vi "xxxx.vi"(8 "error in (no error)":errorcluster, 11 "Context Actor in":refnum<class "Context Actor.lvclass">) -> (0 "error out":errorcluster, 3 "Context Actor out":refnum<class "Context Actor.lvclass">)   [LabVIEW 2021, in "Context Actor.lvlib" / "Context Actor.lvclass"]
uses:
  Context Actor.lvclass
  Context Actor.lvclass/Context Actor.ctl
  Context State/Context State.lvclass
  State Pattern/State Pattern.lvclass
  C:/Program Files/National Instruments/LabVIEW 2021/vi.lib/ActorFramework/Actor/Actor.lvclass
  C:/PPLs/Design-Patterns/State Pattern/Context/Context State/Context State.lvclass
  C:/PPLs/Design-Patterns/State Pattern/State Pattern/State Pattern.lvclass
  C:/PPLs/Design-Patterns/State Pattern/Context Actor/Context Actor.lvclass
  C:/PPLs/Design-Patterns/State Pattern/xxxx/xxxx/xxxx.lvclass
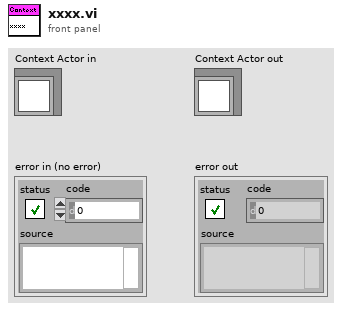
[diagram p1: front panel]
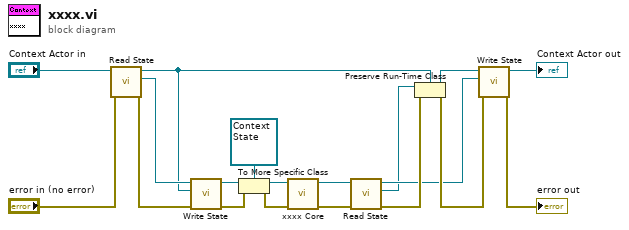
[diagram p0: block diagram]
diagram:
  n1 = call-dynamic "Read State.vi"("error in (no error)"="error in (no error)", "Context Actor in"="Context Actor in") -> ("error out"=w18:errorcluster, "State"=w11:refnum<class "State Pattern.lvclass">, "Context Actor out"=w10:refnum<class "Context Actor.lvclass">)  [unwired: 7 in]
  n2 = call-dynamic "Write State.vi"("error in (no error)"=w18, "State"=w10, "State Pattern in"=w11) -> ("error out"=w6:errorcluster, "State Pattern out"=w9:refnum<class "State Pattern.lvclass">)  [unwired: 7 in]
  n3 = To More Specific Class(target class=refnum<class "Context State.lvclass"> refnum ("Context.lvlib:Context State.lvclass"), reference=w9, error in=w6) -> (specific class reference=w8:refnum<class "Context State.lvclass">, error out=w5:errorcluster)
  n4 = call-dynamic "xxxx Core.vi"("error in (no error)"=w5, "Context State in"=w8) -> ("error out"=w12:errorcluster, "Context State out"=w13:refnum<class "Context State.lvclass">)  [unwired: 8 in]
  n5 = call-dynamic "Read State.vi"("error in (no error)"=w12, "State Pattern in"=w13) -> ("error out"=w17:errorcluster, "State"=w14:refnum<class "State Pattern.lvclass">, "State Pattern out"=w15:refnum<class "Context State.lvclass">)  [unwired: 7 in]
  n6 = Preserve Run-Time Class(object in=w14, error in=w17, 2:w10) -> (object out=w19:refnum<class "Context Actor.lvclass">, error out=w16:errorcluster)
  n7 = call-dynamic "Write State.vi"("error in (no error)"=w16, "State"=w15, "Context Actor in"=w19) -> ("error out"=→"error out":errorcluster, "Context Actor out"=→"Context Actor out":refnum<class "Context Actor.lvclass">)  [unwired: 7 in]
